vi "check ID validity.vi"(8 "error in (no error)":errorcluster, 11 "ID in":string) -> (0 "error out":errorcluster, 3 "ID out":string)   [LabVIEW 2018, in "LV2Julia_core.lvlib"]
uses:
  <vilib>/Utility/error.llb/Error Cluster From Error Code.vi
  <vilib>/regexp/Match Regular Expression.xnode
  <vilib>/ErrorRing/Error Ring.xnode
  LV2Julia_core.lvlib
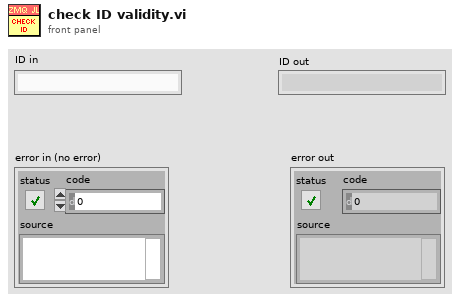
[diagram p1: front panel]
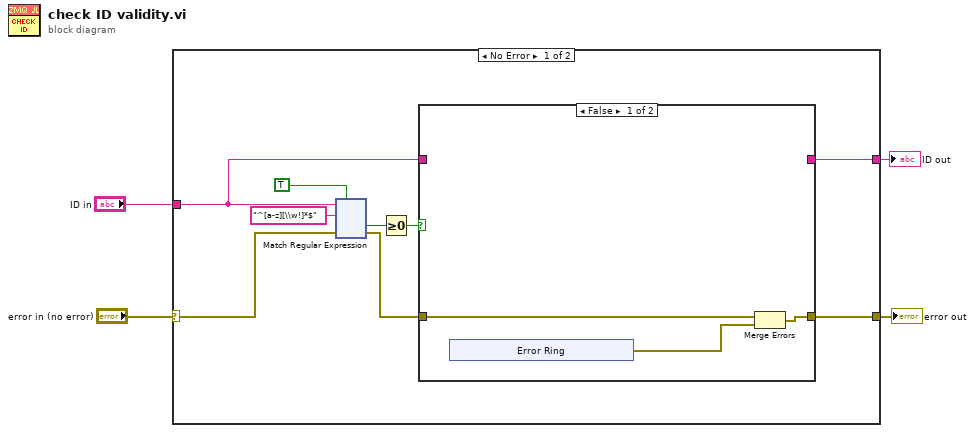
[diagram p0: block diagram]
diagram:
  n1 = case shown="No Error" "error in (no error)" {
    selector: "error in (no error)" -> [w12 w138]
    tunnel: [w13 w138] -> w3
    tunnel: "ID in" -> [w5 _]
    tunnel: [w6 _] -> w1
    frame No Error {
      n2 = xnode "Match Regular Expression"("input string"=w5, "regular expression"="^[a-z][\\w!]*$", "error in"=w12, "ignore case? (F)"=TRUE) -> ("offset past match"=w8:i32, "error out"=w11:errorcluster)  [unwired: 2 in, 3 out]
      n3 = Greater Or Equal To 0?(x=w8) -> (x >= 0?=w7:bool)
      n4 = case shown="False" w7 {
        tunnel: [w16 w23] -> w13
        tunnel: w11 -> [w15 w23]
        tunnel: [_ w22] -> w6
        tunnel: w5 -> [_ w22]
        frame False {
          n5 = xnode "Error Ring"() -> ("error out"=w14:errorcluster)
          n6 = Merge Errors(w15, w14) -> (w16:errorcluster)
        }
        frame True {
        }
      }
    }
    frame Error {
    }
  }
  "error out" <- w3
  "ID out" <- w1
